vi "Old - Gear Line Up.vi"(4 "R/G/B":cluster{"Lower value":i32, "Upper value":i32}[](array[cluster])=[{"Lower value"=0, "Upper value"=40}, {"Lower value"=80, "Upper value"=255}, {"Lower value"=0, "Upper value"=255}], 5 "Camera Image":T1, 6 "Angle Reduction Factor":dbl, 7 "Current Angle":dbl, 8 "Error in":errorcluster, 9 "Encoder Reduction Factor":dbl, 10 "Ref-Nums":T2={"Drive"="RobotDrive", "Gyro"="Gyro", "Talon"="LeftMtr"}, 11 "Auto":bool) -> (0 "Error out":errorcluster)   [LabVIEW 2017]
uses:
  <vilib>/vision/Image Controls.llb/IMAQ Image.ctl
panel:
  out "Image Dimensions":cluster{"X Resolution":i32, "Y Resolution":i32}
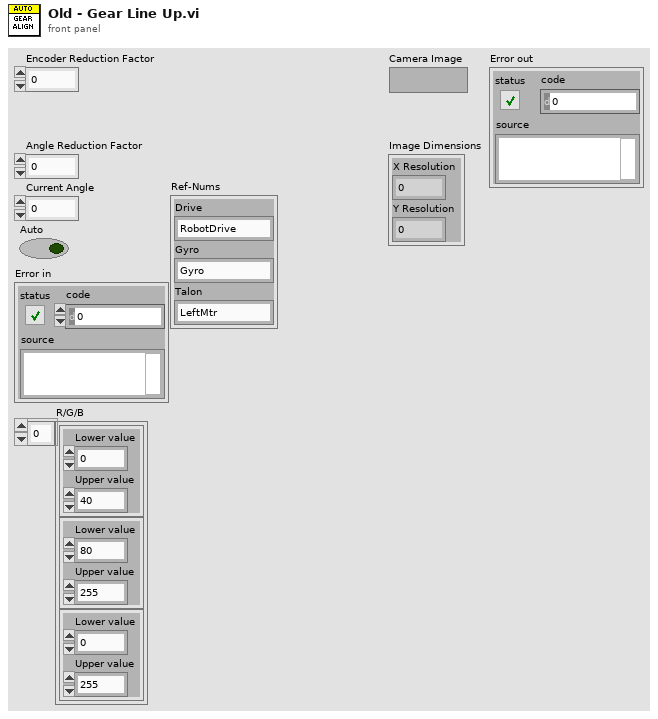
[diagram p1: front panel]
types:
  T1 = typedef "IMAQ Image.ctl" = refnum<image>
  T2 = cluster{"Drive":string, "Gyro":string, "Talon":string}
  T3 = typedef "WPI_RobotDriveDevRef.ctl" = cluster{"DevStatus":errorcluster, "Motors[]":T4[], "Square Inputs":bool, "Max Output":dbl}
  T4 = typedef "WPI_MotorControlDeviceRef.ctl" = cluster{"DeviceStatus":errorcluster, "Type":T5, "PWM":cluster{"PWM Channel":T6, "DeadBand":T7}, "CAN":cluster{"Device Number":u8, "SetOutput VI Ref":variant, "GetOutput VI Ref":variant, "Enable VI Ref":variant, "Disable VI Ref":variant, "Data":variant}, "Invert":bool, "DIO PWM":cluster{"PWM \"Enable\" Channel":T6, "DIOChannel":T8, "PWM Rate":dbl}}
  T5 = typedef "WPI_MotorControlType.ctl" = enum16{"PWM", "CAN", "DIO PWM"}
  T6 = typedef "FPGA_DIOPWMChannel.ctl" = enum8{"PWM 0", "PWM 1", "PWM 2", "PWM 3", "PWM 4", "PWM 5", "PWM 6", "PWM 7", "PWM 8", "PWM 9", "PWM MXP 0", "PWM MXP 1", "PWM MXP 2", "PWM MXP 3", "PWM MXP 4", "PWM MXP 5", "PWM MXP 6", "PWM MXP 7", "PWM MXP 8", "PWM MXP 9", "Invalid"}
  T7 = typedef "WPI_PWMDeadband.ctl" = cluster{"Name":string, "maxPositivePwm":i32, "minPositivePwm":i32, "centerPwm":i32, "maxNegativePwm":i32, "minNegativePwm":i32, "angularRange":u16}
  T8 = typedef "FPGA_DIOChannel.ctl" = enum8{"DIO 0", "DIO 1", "DIO 2", "DIO 3", "DIO 4", "DIO 5", "DIO 6", "DIO 7", "DIO 8", "DIO 9", "DIO MXP 0", "DIO MXP 1", "DIO MXP 2", "DIO MXP 3", "DIO MXP 4", "DIO MXP 5", "DIO MXP 6", "DIO MXP 7", "DIO MXP 8", "DIO MXP 9", "DIO MXP 10", "DIO MXP 11", "DIO MXP 12", "DIO MXP 13", "DIO MXP 14", "DIO MXP 15", "SPI Port CS1", "SPI Port CS2", "SPI Port CS3", "SPI Port MISO", "SPI Port MOSI", "Invalid"}
  T9 = cluster{"Left":dbl, "Top":dbl, "Right":dbl, "Bottom":dbl}
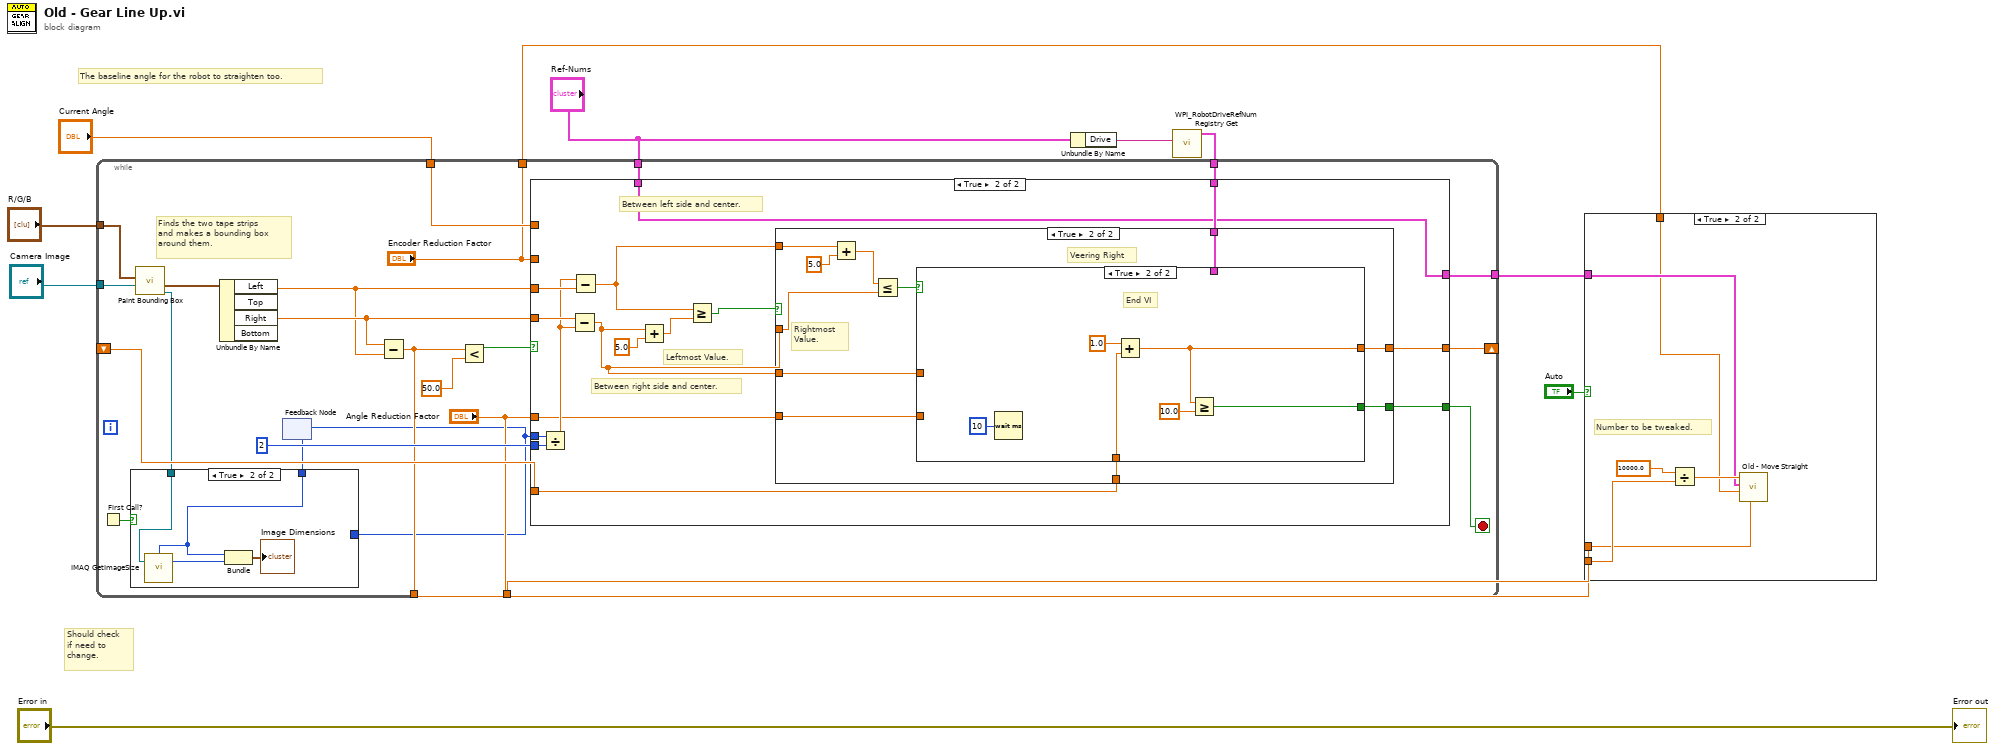
[diagram p0: block diagram]
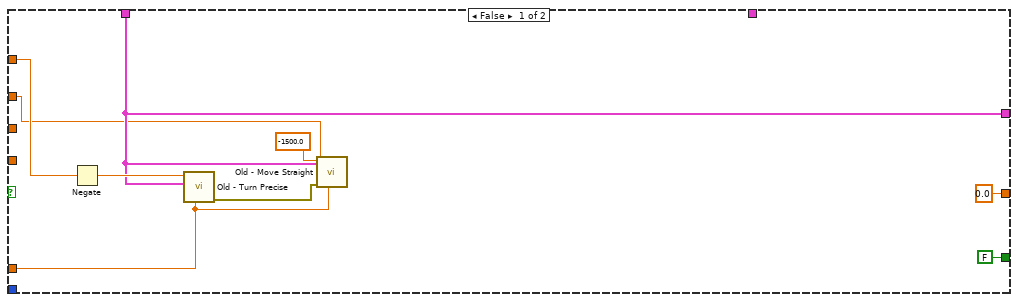
[diagram p4: hidden frame]
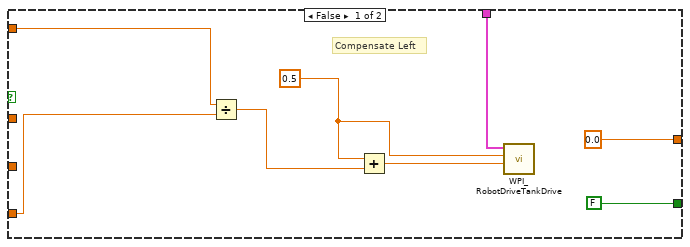
[diagram p5: hidden frame]
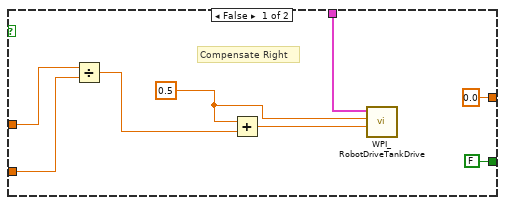
[diagram p6: hidden frame]
diagram:
  # "The baseline angle for the robot to straighten too."
  # "Should check\nif need to\nchange."
  n1 = Unbundle By Name("Ref-Nums") -> ("Drive"=w12:string)
  n2 = call <vilib>:"WPI_RobotDriveRefNum Registry Get.vi"("refnum name"=w12) -> ("RobotDriveDevRef"=w11:T3)  [unwired: 9 in, 1 out]
  n3 = while {
    tunnel: w11 -> [w33]
    shift-right: [w32] -> _
    shift-left: _ -> [w31]
    tunnel: "Current Angle" -> [w24]
    tunnel: [w23] -> w9
    tunnel: "Ref-Nums" -> [w22]
    tunnel: [w21] -> w4
    tunnel: ["Angle Reduction Factor"] -> w6
    tunnel: ["Encoder Reduction Factor"] -> w5
    tunnel: "Camera Image" -> [w14]
    tunnel: "R/G/B" -> [w13]
    stop <- w30 stop-if-true
    # "Finds the two tape strips\nand makes a bounding box\naround them."
    n4 = First Call?() -> (First Call?: T/F=w18:bool)
    n5 = call "Paint Bounding Box.vi"("Camera Image"=w14, 10:w13) -> ("Thresholded Image"=w17:T1, "Bounding Box Final"=w34:T9)  [unwired: 5 in, 3 out]
    n6 = Unbundle By Name(w34) -> ("Left"=w27:dbl, "Right"=w28:dbl)  [unwired: 2 out]
    n7 = feedback #1() -> (w15:i32)  [unwired: 1 in]
    n8 = case shown="True" w18 {
      tunnel: [w35 w37] -> w16
      tunnel: w17 -> [_ w36]
      tunnel: w15 -> [w35 _]
      frame False {
      }
      frame True {
        n9 = call "IMAQ GetImageSize"("Image"=w36) -> ("Y Resolution"=w38:i32, "X Resolution"=w37:i32)  [unwired: 3 in, 1 out]
        n10 = Bundle("X Resolution"=w37, "Y Resolution"=w38) -> (→"Image Dimensions":cluster{"X Resolution":i32, "Y Resolution":i32})  [unwired: 1 in]
      }
    }
    n11 = feedback-in #1(w16) -> ()
    n12 = Subtract(x=w28, y=w27) -> (x-y=w21:dbl)
    n13 = Less?(x=w21, y=50.0) -> (x < y?=w25:bool)
    n14 = case shown="True" w25 {
      tunnel: w33 -> [_ w63]
      tunnel: [0.0 w62] -> w32
      tunnel: w31 -> [_ w61]
      tunnel: [FALSE w60] -> w30
      tunnel: w15 -> [_ w59]
      tunnel: 2 ("y") -> [_ w58]
      tunnel: w28 -> [_ w57]
      tunnel: w27 -> [_ w56]
      tunnel: w24 -> [w44 _]
      tunnel: [w42 w50] -> w23
      tunnel: w22 -> [w42 w50]
      tunnel: "Angle Reduction Factor" -> [w41 w49]
      tunnel: "Encoder Reduction Factor" -> [w40 _]
      frame False {
        n15 = Negate(x=w44) -> (-x=w43:dbl)
        n16 = call "Old - Turn Precise.vi"("Angle Reduction Factor"=w41, "Ref-Nums"=w42, "Angle"=w43) -> ("error out"=w45:errorcluster)  [unwired: 8 in]
        n17 = call "Old - Move Straight.vi"("Angle Reduction Factor"=w41, "error in (no error)"=w45, "Encoder Reduction Factor"=w40, "Ref-Nums"=w42, "Encoder Distance"=-1500.0) -> ()  [unwired: 6 in, 1 out]
      }
      frame True {
        # "Between right side and center."
        # "Leftmost Value."
        # "Between left side and center."
        n18 = Divide(x=w59, y=w58) -> (x/y=w55:dbl)
        n19 = Subtract(x=w57, y=w55) -> (x-y=w52:dbl)
        n20 = Subtract(x=w55, y=w56) -> (x-y=w54:dbl)
        n21 = Add(x=w52, y=5.0) -> (x+y=w53:dbl)
        n22 = Greater Or Equal?(x=w54, y=w53) -> (x >= y?=w64:bool)
        n23 = case shown="True" w64 {
          tunnel: w63 -> [w70 w82]
          tunnel: w54 -> [w72 w74]
          tunnel: w49 -> [w71 w81]
          tunnel: [0.0 w80] -> w62
          tunnel: w61 -> [_ w79]
          tunnel: [FALSE w78] -> w60
          tunnel: w52 -> [_ w77]
          tunnel: w52 -> [_ w76]
          frame False {
            w65 = 0.5
            # "Compensate Left"
            n24 = Divide(x=w72, y=w71) -> (x/y=w66:dbl)
            n25 = Add(x=w65, y=w66) -> (x+y=w67:dbl)
            n26 = call <vilib>:"WPI_RobotDriveTankDrive.vi"("Right axis value"=w67, "Left axis value"=w65, "RobotDriveDevRef"=w70) -> ()  [unwired: 6 in, 3 out]
          }
          frame True {
            # "Rightmost \nValue."
            # "Veering Right"
            n27 = Add(x=w74, y=5.0) -> (x+y=w73:dbl)
            n28 = Less Or Equal?(x=w73, y=w76) -> (x <= y?=w83:bool)
            n29 = case shown="True" w83 {
              tunnel: w82 -> [w91 _]
              tunnel: w81 -> [w90 _]
              tunnel: [0.0 w94] -> w80
              tunnel: w79 -> [_ w95]
              tunnel: [FALSE w92] -> w78
              tunnel: w77 -> [w84 _]
              frame False {
                w85 = 0.5
                # "Compensate Right"
                n30 = Divide(x=w84, y=w90) -> (x/y=w86:dbl)
                n31 = Add(x=w85, y=w86) -> (x+y=w87:dbl)
                n32 = call <vilib>:"WPI_RobotDriveTankDrive.vi"("Right axis value"=w87, "Left axis value"=w85, "RobotDriveDevRef"=w91) -> ()  [unwired: 6 in, 3 out]
              }
              frame True {
                # "End VI"
                n33 = Wait (ms)(milliseconds to wait=u32 10) -> ()  [unwired: 1 out]
                n34 = Add(x=1.0 ("y"), y=w95) -> (x+y=w94:dbl)
                n35 = Greater Or Equal?(x=w94, y=10.0) -> (x >= y?=w92:bool)
              }
            }
          }
        }
      }
    }
  }
  n36 = case shown="True" "Auto" {
    tunnel: w4 -> [_ w103]
    tunnel: w9 -> [_ w100]
    tunnel: w6 -> [_ w99]
    tunnel: w5 -> [_ w98]
    frame False {
    }
    frame True {
      # "Number to be tweaked."
      n37 = Divide(x=10000.0, y=w103) -> (x/y=w101:dbl)
      n38 = call "Old - Move Straight.vi"("Angle Reduction Factor"=w99, "Encoder Reduction Factor"=w98, "Ref-Nums"=w100, "Encoder Distance"=w101) -> ()  [unwired: 7 in, 1 out]
    }
  }
  "Error out" <- "Error in"
